vi "BounceFrequency.vi"() -> ()   [LabVIEW 2018]
uses:
  <vilib>/Analysis/NI_AALPro.lvlib
panel:
  in  "hex scale":dbl=25.0 format="%#_13g"
  in  "invert":bool
  in  "stop":bool
  in  "XY Graph 2":cluster{"z (mm)":dbl[], "B (T)":dbl[]}[](graph)=[{"z (mm)"=array[861 elements], "B (T)"=array[861 elements]}, {"z (mm)"=array[2601 elements], "B (T)"=array[2601 elements]}]
  out "Bounce Freq (Hz)":dbl=4419788.9496182045 format="%_3p"
  out "Polynomial Coefficients":dbl[](array[numeric])=[0.00029459058298819587, 0.04992791549088847, 7.015442904616151, 0.6152992958501168, 8.46385495190754, 4.478538559917406, -6.166749014549826]
  in  "polynomial order":i32=6
  out "XY Graph":cluster{dbl[], "Best Polynomial Fit":dbl[]}[](graph)=[{[-0.024450000000000027, -0.023840000000000028, -0.02323000000000003, -0.02262000000000003, -0.02201000000000003, -0.02140000000000003, -0.02078000000000002, -0.02017000000000002, -0.019560000000000022, -0.018950000000000022, -0.018340000000000023, -0.017730000000000024, -0.017120000000000024, -0.016500000000000015, -0.015890000000000015, -0.015280000000000016, -0.014670000000000016, -0.014060000000000017, -0.013450000000000017, -0.012840000000000018, -0.012230000000000019, -0.01161000000000001, -0.01100000000000001, -0.01039000000000001, -0.009780000000000011, -0.009170000000000011, -0.008560000000000012, -0.007950000000000013, -0.007330000000000003, -0.006720000000000004, -0.006110000000000004, -0.005500000000000005, -0.0048900000000000055, -0.004280000000000006, -0.0036700000000000066, -0.003060000000000007, -0.0024399999999999977, -0.0018299999999999983, -0.0012199999999999989, -0.0006099999999999994, 0.0, 0.0006099999999999994, 0.0012199999999999989, 0.0018400000000000083, 0.0024500000000000077, 0.003060000000000007, 0.0036700000000000066, 0.004280000000000006, 0.0048900000000000055, 0.005500000000000005, 0.006120000000000014, 0.006730000000000014, 0.007340000000000013, 0.007950000000000013, 0.008560000000000012, 0.009170000000000011, 0.009780000000000011, 0.01039000000000001, 0.01101000000000002, 0.01162000000000002, 0.012230000000000019, 0.012840000000000018, 0.013450000000000017, 0.014060000000000017, 0.014670000000000016, 0.01528999999999997, 0.01589999999999997, 0.01650999999999997, 0.01711999999999997, 0.017730000000000024, 0.018340000000000023, 0.018950000000000022, 0.019560000000000022, 0.020179999999999976, 0.020789999999999975, 0.021399999999999975, 0.022009999999999974], "Best Polynomial Fit"=[2.9283553031730007, 2.7880280691170003, 2.6480582837652005, 2.5085480913732003, 2.371240088592801, 2.2373815517253, 2.107045434413301, 1.980125601357701, 1.8566598345576013, 1.7366999549739006, 1.6202030772151002, 1.507180630143301, 1.3976087058564004, 1.2924559096882007, 1.1916730220641, 1.095299131585, 1.003258821647401, 0.9156588702495005, 0.832388795996601, 0.7535591803192014, 0.6790682484510007, 0.6089391251583005, 0.5432676013808004, 0.4815154429736008, 0.42368264588430105, 0.36971609319710064, 0.31971890317830054, 0.2736183858595709, 0.2314068032105001, 0.19314804325791135, 0.15874649568020072, 0.12783027942114078, 0.10023433441531004, 0.07602906699289047, 0.055143878824140735, 0.037611368535061196, 0.023433379499301132, 0.012608348047300488, 0.0051531158146200795, 0.0010493703296114987, 0.0, 0.002333624705480375, 0.008084931609170454, 0.01726292318307099, 0.02985740946171056, 0.04588458110151006, 0.06527674457935984, 0.08805159309142052, 0.11428693310473026, 0.14406845129161994, 0.17820744689661083, 0.21670991351604085, 0.2596700128831304, 0.3069922101345708, 0.3586384781337606, 0.41472878267730007, 0.47524468543519127, 0.5400741864108305, 0.6098477170301706, 0.6859584451647103, 0.7685123676040702, 0.8574639565229307, 0.9527647429171004, 1.0544951958233848, 1.1626248119719782, 1.2772000566330095, 1.398107333569194, 1.5263224217990867, 1.6635176629404604, 1.8095359227933652, 1.9645928045873848, 2.1285580050928914, 2.301461530706522, 2.4833884044680747, 2.6740886004247155, 2.8739624173624803, 3.084204788507761]}, {[-0.024450000000000027, -0.023840000000000028, -0.02323000000000003, -0.02262000000000003, -0.02201000000000003, -0.02140000000000003, -0.02078000000000002, -0.02017000000000002, -0.019560000000000022, -0.018950000000000022, -0.018340000000000023, -0.017730000000000024, -0.017120000000000024, -0.016500000000000015, -0.015890000000000015, -0.015280000000000016, -0.014670000000000016, -0.014060000000000017, -0.013450000000000017, -0.012840000000000018, -0.012230000000000019, -0.01161000000000001, -0.01100000000000001, -0.01039000000000001, -0.009780000000000011, -0.009170000000000011, -0.008560000000000012, -0.007950000000000013, -0.007330000000000003, -0.006720000000000004, -0.006110000000000004, -0.005500000000000005, -0.0048900000000000055, -0.004280000000000006, -0.0036700000000000066, -0.003060000000000007, -0.0024399999999999977, -0.0018299999999999983, -0.0012199999999999989, -0.0006099999999999994, 0.0, 0.0006099999999999994, 0.0012199999999999989, 0.0018400000000000083, 0.0024500000000000077, 0.003060000000000007, 0.0036700000000000066, 0.004280000000000006, 0.0048900000000000055, 0.005500000000000005, 0.006120000000000014, 0.006730000000000014, 0.007340000000000013, 0.007950000000000013, 0.008560000000000012, 0.009170000000000011, 0.009780000000000011, 0.01039000000000001, 0.01101000000000002, 0.01162000000000002, 0.012230000000000019, 0.012840000000000018, 0.013450000000000017, 0.014060000000000017, 0.014670000000000016, 0.01528999999999997, 0.01589999999999997, 0.01650999999999997, 0.01711999999999997, 0.017730000000000024, 0.018340000000000023, 0.018950000000000022, 0.019560000000000022, 0.020179999999999976, 0.020789999999999975, 0.021399999999999975, 0.022009999999999974], "Best Polynomial Fit"=[2.928150730708582, 2.7870327568027675, 2.6472135862488844, 2.5091472506825014, 2.373241381969, 2.2398597543506926, 2.1072102075423946, 1.979858796780168, 1.8558881437480728, 1.735510354277118, 1.6189055862219752, 1.5062242556043903, 1.3975891869085681, 1.291419697362094, 1.1912153073300822, 1.0952814595353662, 1.0036506935730893, 0.9163379014651477, 0.8333421419518816, 0.7546483989357305, 0.6802292840768676, 0.6089311906196195, 0.5430060942141358, 0.4812144616290009, 0.42349523622832713, 0.36978268726014435, 0.3200077764483323, 0.2740994687365253, 0.23132681633735622, 0.19299729551696326, 0.15832043822184427, 0.12722926556017816, 0.09966053430364802, 0.0755557116276449, 0.05486189400344564, 0.037532670242363834, 0.023326878456241054, 0.012671354551664921, 0.0052876484215423365, 0.0011629906040369154, 0.00029459058298819587, 0.0026901638283618316, 0.008368402988673218, 0.017534603179654284, 0.02993559063860269, 0.04574604462403128, 0.06503236491027747, 0.08787344937343167, 0.11436082918006019, 0.14459874812790136, 0.17929622108444102, 0.2174655409787048, 0.25977680002739456, 0.30638497193758013, 0.3574572982882705, 0.41317303186741033, 0.4737231241608471, 0.5393098569932749, 0.6113526484585128, 0.6877542999956605, 0.7698668053650941, 0.8579331143862753, 0.9522048166201686, 1.0529414370064838, 1.16040967565289, 1.2768191065284122, 1.3986969911120397, 1.5281458790923657, 1.6654525022937017, 1.8109061114285563, 1.964797379883091, 2.1274172516546903, 2.2990557334413673, 2.4830460711526543, 2.6737412367546205, 2.874311023261134, 3.0850283761415898]}]
  # "To get your potentials in here,, go into the potential editor, right click and select Copy Data\nthen right click on the top graph here and select Data Operations--Paste Data"
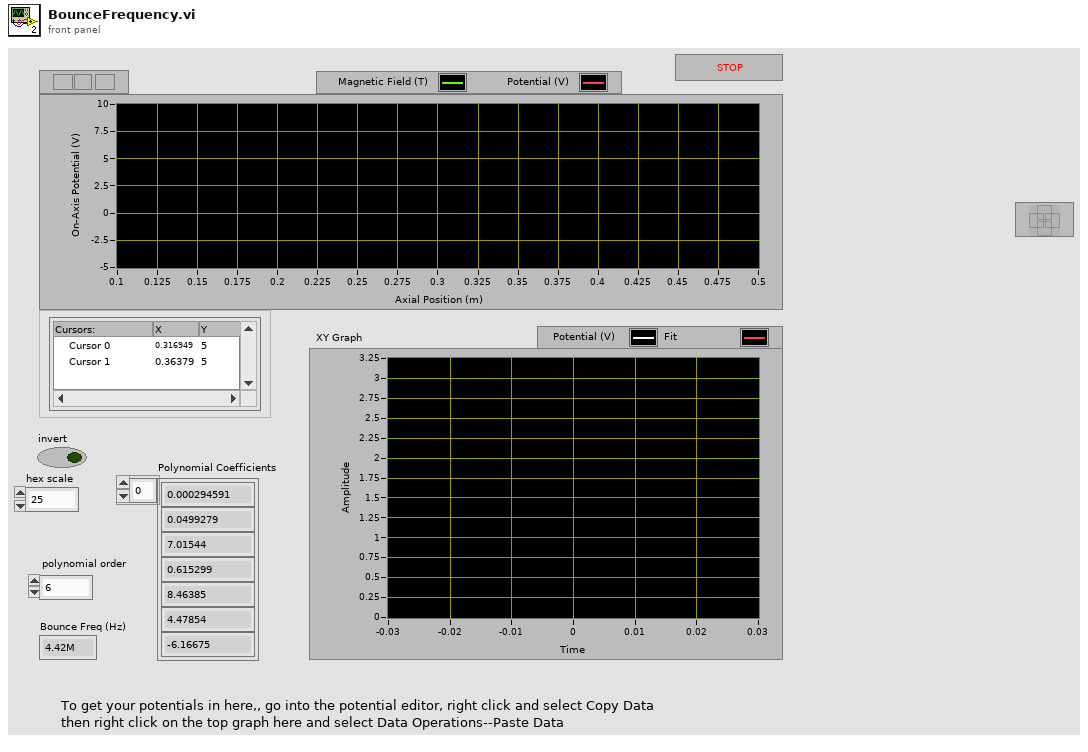
[diagram p1: front panel]
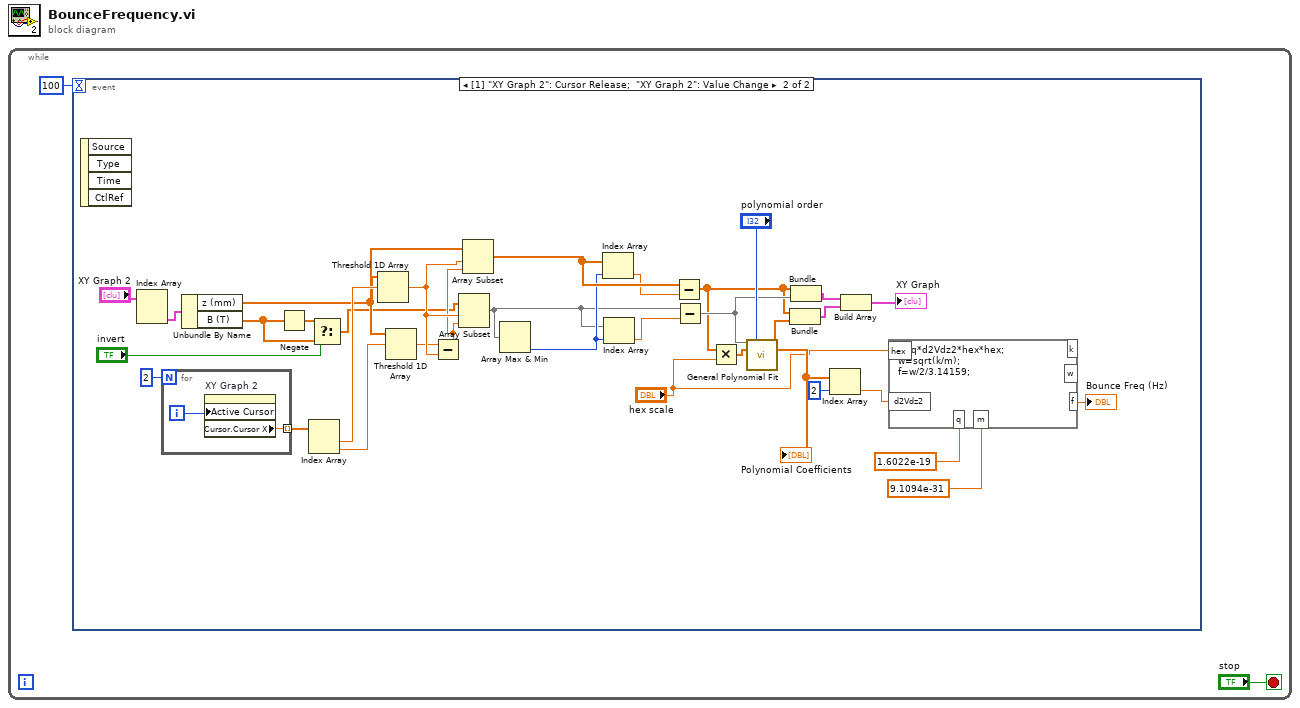
[diagram p0: block diagram]
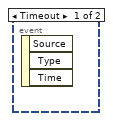
[diagram p2: hidden frame]
diagram:
  n1 = while {
    stop <- "stop" stop-if-true
    n2 = event shown="[1] \"XY Graph 2\": Cursor Release;  \"XY Graph 2\": Value Change" {
      selector: _ -> [_ _]
      dyn-events: _ -> [_ _]
      timeout: 100 -> [_ _]
      event Timeout {
        n3 = event-data() -> ()  [unwired: 1 in, 3 out]
      }
      event "XY Graph 2": Cursor Release; "XY Graph 2": Value Change {
        n4 = event-data() -> ()  [unwired: 1 in, 4 out]
        n5 = Index Array(array="XY Graph 2") -> (element #2=w36:cluster{"z (mm)":dbl[], "B (T)":dbl[]})  [unwired: 2 in, 1 out]
        n6 = for {
          N: 2 -> [_]
          tunnel: [w37] -> w32 mode=indexing
          i -> [w38]
          n7 = property on="XY Graph 2" class="XYGraph (strict)"("Active Cursor"=w38) -> ("Cursor.Cursor X"=w37:dbl)  [unwired: 2 in, 2 out]
        }
        n8 = Unbundle By Name(w36) -> ("z (mm)"=w29:dbl[], "B (T)"=w8:dbl[])
        n9 = Negate(x=w8) -> (-x=w9:dbl[])
        n10 = Index Array(array=w32) -> (element #1=w33:dbl, element #2=w34:dbl)  [unwired: 2 in]
        n11 = Select(t=w9, s="invert", f=w8) -> (s? t:f=w7:dbl[])
        n12 = Threshold 1D Array(2:w33, 3:w29) -> (0:w35:dbl)  [unwired: 1 in]
        n13 = Threshold 1D Array(2:w34, 3:w29) -> (0:w31:dbl)  [unwired: 1 in]
        n14 = Subtract(x=w31, y=w35) -> (x-y=w30:dbl)
        n15 = Array Subset(array=w7, index=w35, length=w30) -> (w10:dbl[])
        n16 = Array Subset(array=w29, index=w35, length=w30) -> (w14:dbl[])
        n17 = Array Max & Min(array=w10) -> (min index (indices)=w12:i32)  [unwired: 3 out]
        n18 = Index Array(array=w14, index=w12) -> (element=w13:dbl)
        n19 = Index Array(array=w10, index=w12) -> (element=w11:dbl)
        n20 = Subtract(x=w14, y=w13) -> (x-y=w4:dbl[])
        n21 = Subtract(x=w10, y=w11) -> (x-y=w19:dbl[])
        n22 = Multiply(x=w4, y="hex scale") -> (x*y=w5:dbl[])
        n23 = call <vilib>:"General Polynomial Fit.vi"("Y"=w19, "polynomial order"="polynomial order", "X"=w5) -> ("Best Polynomial Fit"=w21:dbl[], "Polynomial Coefficients"=w25:dbl[])  [unwired: 9 in, 2 out]
        "Polynomial Coefficients" <- w25
        n24 = Bundle(w4, "Best Polynomial Fit"=w21) -> (w23:cluster{dbl[], "Best Polynomial Fit":dbl[]})  [unwired: 1 in]
        n25 = Bundle(w4, w19) -> (w22:cluster{dbl[], dbl[]})  [unwired: 1 in]
        n26 = Index Array(array=w25, index=2) -> (element=w26:dbl)
        n27 = Build Array(w22, w23) -> (→"XY Graph":cluster{dbl[], "Best Polynomial Fit":dbl[]}[])
        n28 = formula code="k=q*d2Vdz2*hex*hex;\nw=sqrt(k/m);\nf=w/2/3.14159;"("q"=1.6022e-19 ("input variable"), "m"=9.1094e-31 ("input variable"), "d2Vdz2"=w26, "hex"="hex scale") -> ("f"=→"Bounce Freq (Hz)":dbl)  [unwired: 2 out]
      }
    }
  }
